vi "Demo.vi"() -> ()   [LabVIEW 2021]
doc: "本VI是为《我和LabVIEW》一书编写的示例。\n关于本书的介绍请参考网页：\nhttp://ruanqizhen.spaces.live.com/blog/cns!5852D4F797C53FB6!4310.entry"
uses:
  List/List.lvclass
panel:
  out "data":dbl[](array[numeric])
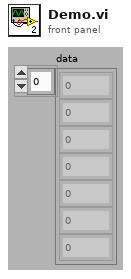
[diagram p1: front panel]
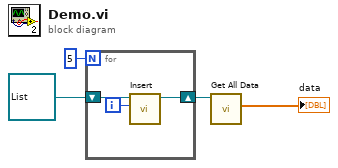
[diagram p0: block diagram]
diagram:
  n1 = for {
    N: 5 -> [_]
    shift-right: [w5] -> w3
    shift-left: refnum<class "List.lvclass"> refnum ("List Node.lvclass") -> [w7]
    i -> [w6]
    n2 = call-dynamic "Insert.vi"("data"=w6, "List Node in"=w7) -> ("List Node out"=w5:refnum<class "List.lvclass">)  [unwired: 1 in, 8 out]
  }
  n3 = call-dynamic "Get All Data.vi"("List in"=w3) -> ("data"=→"data":dbl[])  [unwired: 1 in, 9 out]
